vi "IOC_LV_Panel1.vi"() -> ()   [LabVIEW 2016]
uses:
  <vilib>/Utility/miscctls.llb/LVPointTypeDef.ctl
  <vilib>/Instr/_visa.llb/VISA Configure Serial Port (Instr).vi
panel:
  in  "Boolean":bool
  in  "Baud rate":u64=230400
  in  "COM Port":refnum<visa-resource-name>
  in  "ms":i32=50
  in  "Analog Input Gain":u8 format="%.0b"
  in  "New Address":u8=170
  in  "set Address":bool
  in  "set sn":bool
  in  "New S/N":u32 format="%08x"
  out "S/N":u32 format="%08x"
  out "CPU Clock":u32=170 caption="Clock" format="%.0f [sec]"
  in  "Address":u8=170
  out "value 2":u8=170 caption="value"
  in  "index 2":u8=99 caption="index[0..99]" max=99 step=1
  in  "set scratch":bool
  in  "value":u8=170
  in  "index[0..99]":u8=99 max=99
  out "disable?":bool
  out "gui_refresh":bool
  in  "DigTimeout":u16=170 caption="Digital Timeout[sec]"
  in  "DIGITAL_IO":T1={"DIG_PORT_0 [0..7] (P4)"=[FALSE, FALSE, FALSE, FALSE, FALSE, FALSE, FALSE, FALSE], "DIG_PORT_1 [8..15] (P5)"=[FALSE, FALSE, FALSE, FALSE, FALSE, FALSE, FALSE, FALSE], "DIG_PORT_2 [16..23]  (P3)"=[FALSE, FALSE, FALSE, FALSE, FALSE, FALSE, FALSE, FALSE], "DIG_PORT_3  [24..31]  (P2)"=[FALSE, FALSE, FALSE, FALSE, FALSE, FALSE, FALSE, FALSE], "DIG_PORT_4   [32..39]  (P6)"=[FALSE, FALSE, FALSE, FALSE, FALSE, FALSE, FALSE, FALSE], "DIG_PORT_5  [40..47]  (P7)"=[FALSE, FALSE, FALSE, FALSE, FALSE, FALSE, FALSE, FALSE]} caption="Digital In/Out"
  in  "scan":bool
  in  "Table Control":string[][](table)
  out "user msg":string
  out "Chart":T2(graph)
  in  "AOUT0[%]":dbl(knob) scale=0.0..100.0
  in  "AOUT1[%]":dbl(knob) scale=0.0..100.0
  in  "counter":i32
  in  "stop":bool
  # "Module Setup"
  # "Module Setup"
  # "Virtual Address Setup"
  # "Read Module Data"
  # "Serial Number Setup"
  # "Get Scratch Memory"
  # "Set Scratch Memory"
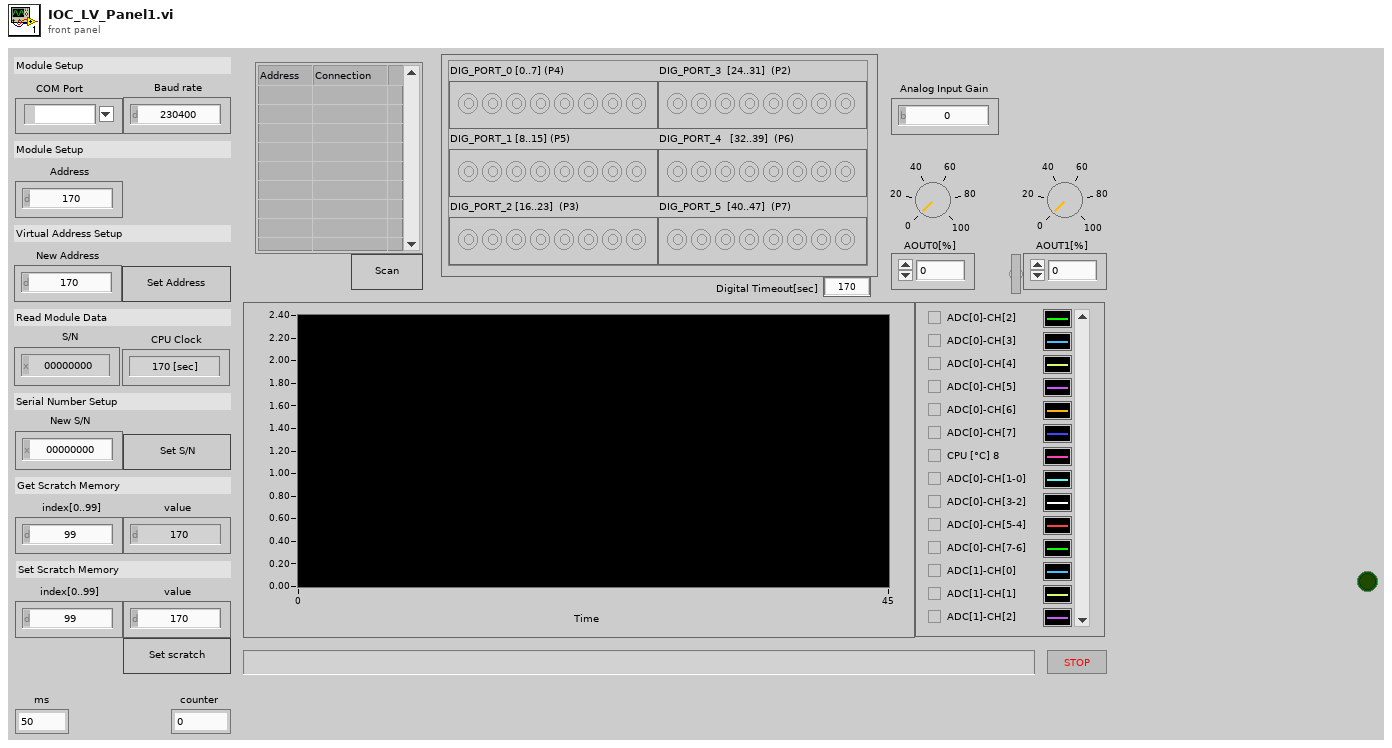
[diagram p1: front panel]
types:
  T1 = cluster{"DIG_PORT_0 [0..7] (P4)":bool[], "DIG_PORT_1 [8..15] (P5)":bool[], "DIG_PORT_2 [16..23]  (P3)":bool[], "DIG_PORT_3  [24..31]  (P2)":bool[], "DIG_PORT_4   [32..39]  (P6)":bool[], "DIG_PORT_5  [40..47]  (P7)":bool[]}
  T2 = cluster{"[0]":sgl, "[1]":sgl, "[2]":sgl, "[3]":sgl, "[4]":sgl, "[5]":sgl, "[6]":sgl, "[7]":sgl, "[8]":sgl, "[9]":sgl, "[10]":sgl, "[11]":sgl, "[12]":sgl, "[13]":sgl, "[14]":sgl, "[15]":sgl, "[16]":sgl, "[17]":sgl, "[18]":sgl, "[19]":sgl, "[20]":sgl}
  T3 = typedef "LVPointTypeDef.ctl" = cluster{"Horizontal":i16, "Vertical":i16}
  T4 = cluster{"ADDRESS":u8, "AOUT CHANNEL":u8, "AOUT value":u16}
  T5 = cluster{"ADDRESS[0.255]":u8, "AIN CHANNEL[0..7]":u8, "gain":u8}
  T6 = cluster{"DIG_PORT_0 [0..7] (P4)":bool[], "DIG_PORT_1 [8..15] (P5)":bool[], "DIG_PORT_2 [16..23]  (P3)":bool[], "DIG_PORT_3  [23..31]  (P2)":bool[], "DIG_PORT_4   [32..39]  (P6)":bool[], "DIG_PORT_5  [40..47]  (P7)":bool[]}
  T7 = cluster{"Address":u8, "index of element":i32, i16, "DigTimeout":u16}
  T8 = cluster{"Address":u8, i32, i16, "DigTimeout":u16}
  T9 = typedef "lveventtype.ctl" = enum32{"Null", "Timeout", "Annotation Menu Selection", "Annotation Menu Selection?", "App Instance Close", "App Instance Close?", "Autoscale Range Change", "Bookmark Info Change", "Cell Edit", "Cell Edit?", "Cursor Grab", "Cursor Grab?", "Cursor Menu Selection", "Cursor Menu Selection?", "Cursor Move", "Cursor Release", "Data Change", "Direction Change", "Display State Change", "Drag Ended", "Drag Enter", "Drag Leave", "Drag Over", "Drag Source Update", "Drag Starting", "Drag Starting?", "Drop", "Exec State Change", "Key Down", "Key Down?", "Key Repeat", "Key Repeat?", "Key Up", "Listbox Double Click", "Menu Activation?", "Menu Selection (App)", "Menu Selection? (App)", "Menu Selection (User)", "Mouse Down", "Mouse Down?", "Mouse Enter", "Mouse Leave", "Mouse Move", "Mouse Up", "Mouse Wheel", "NI Security User Change (App)", "Pane Size", "Panel Close", "Panel Close?", "Panel Resize", "Plot Attribute Change", "Scale Range Change", "Shortcut Menu Activation?", "Shortcut Menu Selection (App)", "Shortcut Menu Selection? (App)", "Shortcut Menu Selection (User)", "Tree Double Click", "Tree Drag", "Tree Drag?", "Tree Drop", "Tree Drop?", "Tree Item Close", "Tree Item Close?", "Tree Item Open", "Tree Item Open?", "User Event", "Value Change"}
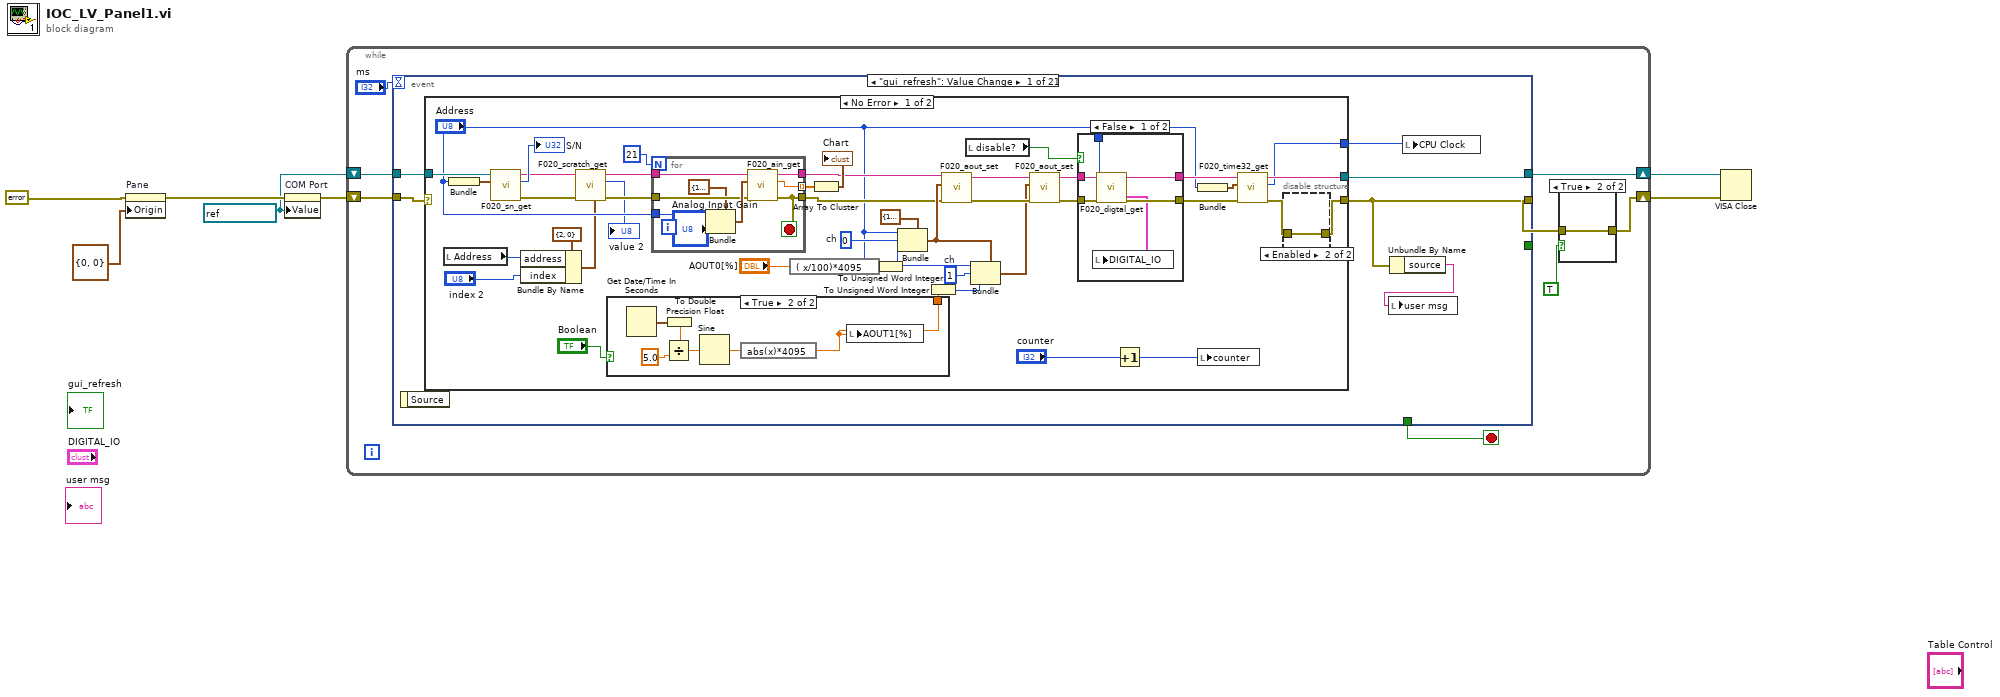
[diagram p0: block diagram]
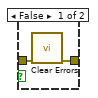
[diagram p2: hidden frame]
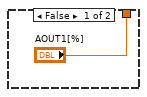
[diagram p3: hidden frame]
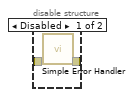
[diagram p4: hidden frame]
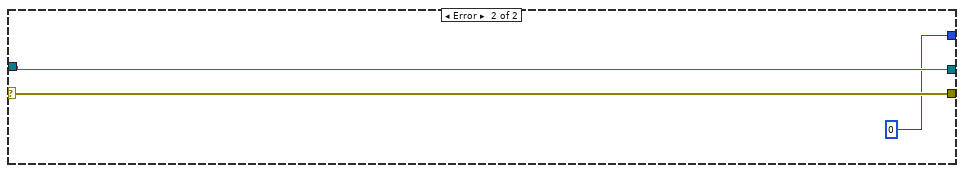
[diagram p6: hidden frame]
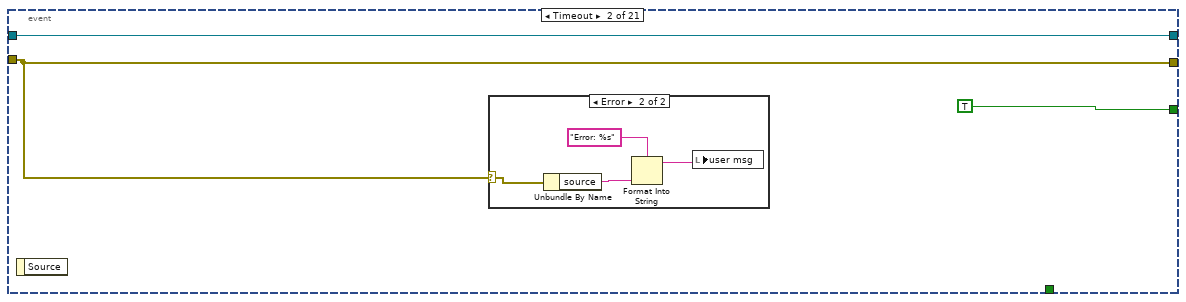
[diagram p7: hidden frame]
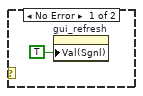
[diagram p8: hidden frame]
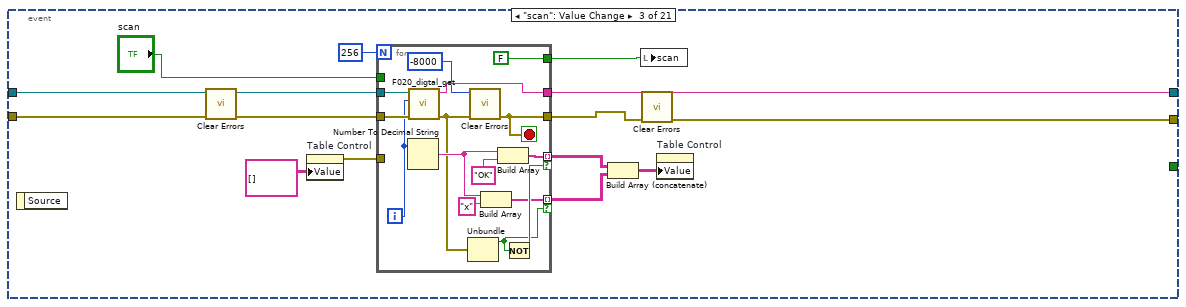
[diagram p9: hidden frame]
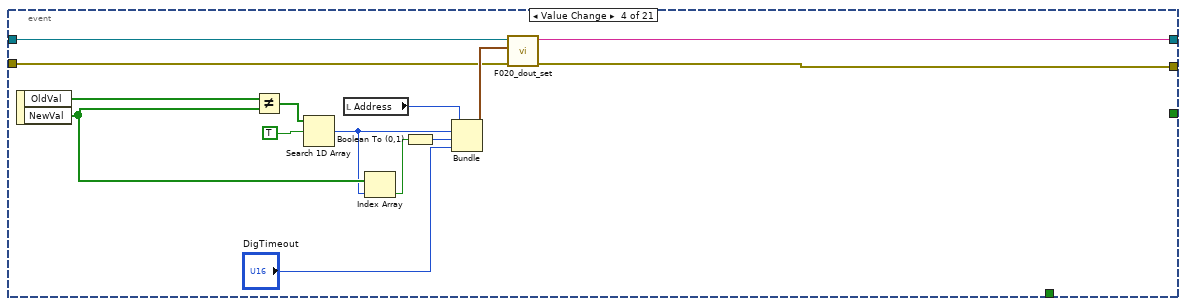
[diagram p10: hidden frame]
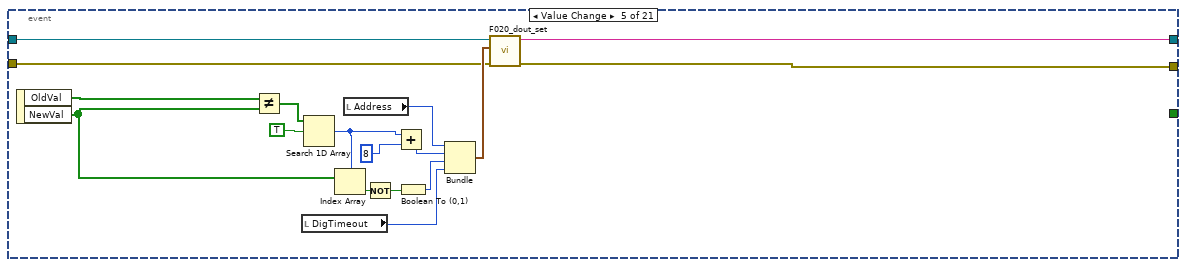
[diagram p11: hidden frame]
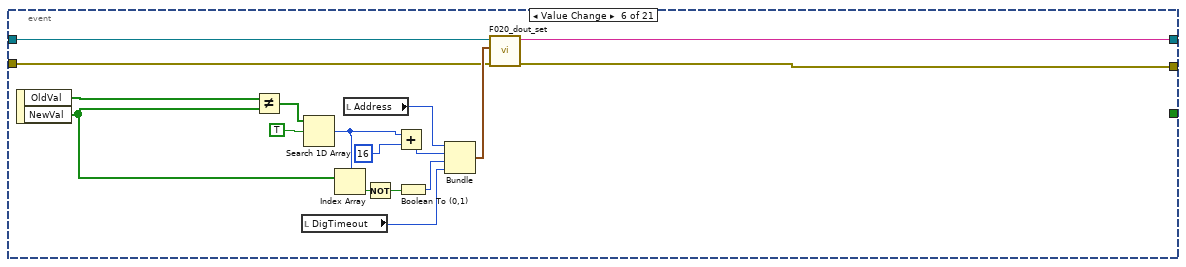
[diagram p12: hidden frame]
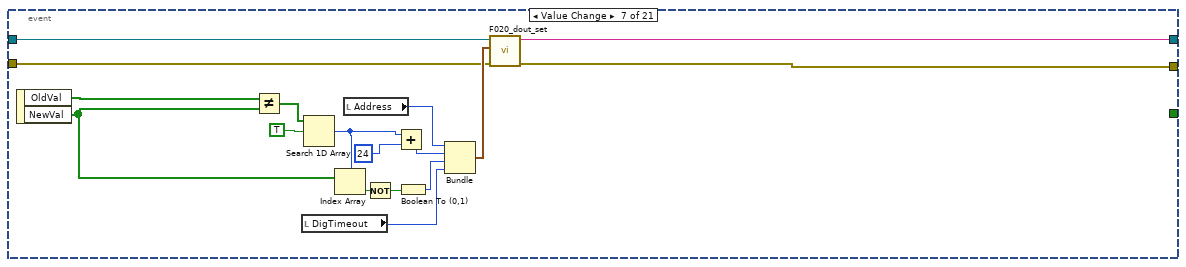
[diagram p13: hidden frame]
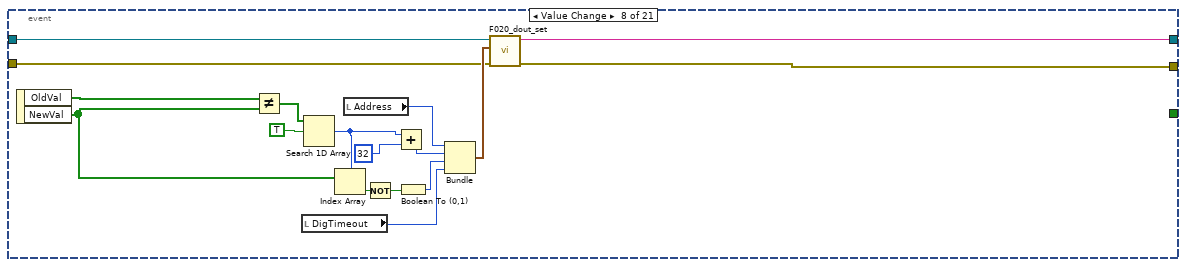
[diagram p14: hidden frame]
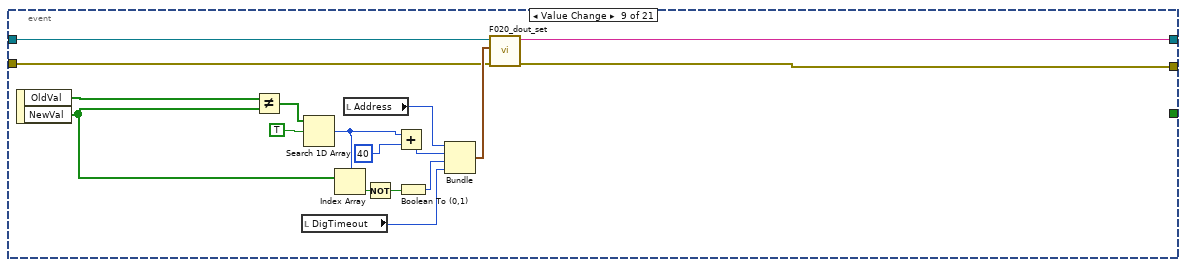
[diagram p15: hidden frame]
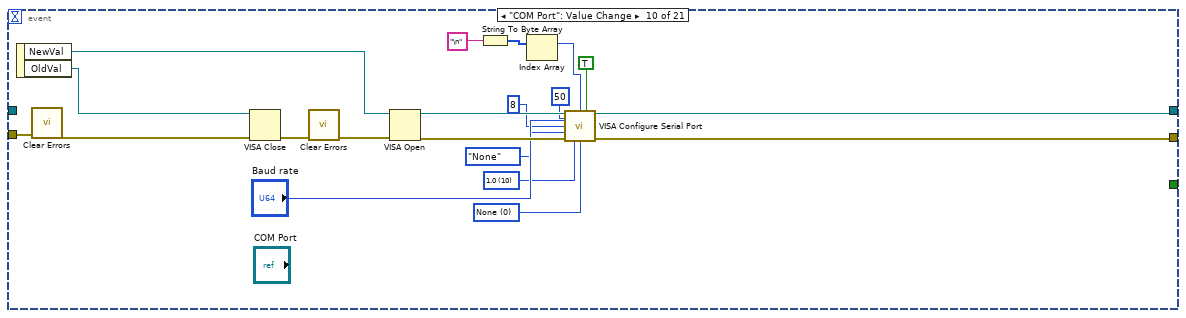
[diagram p16: hidden frame]
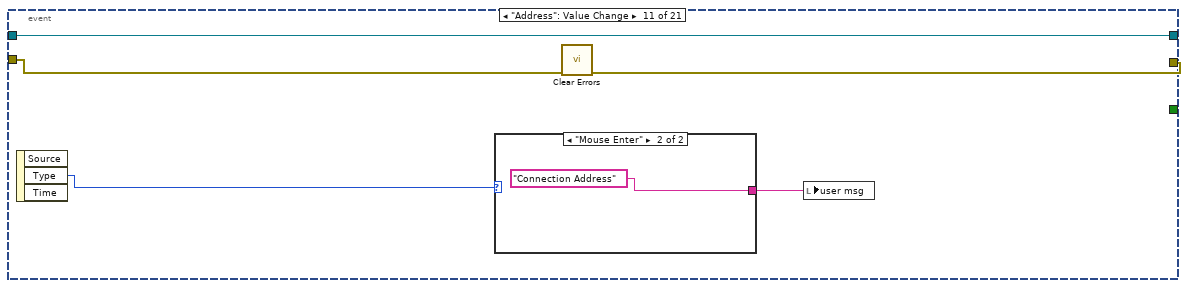
[diagram p17: hidden frame]
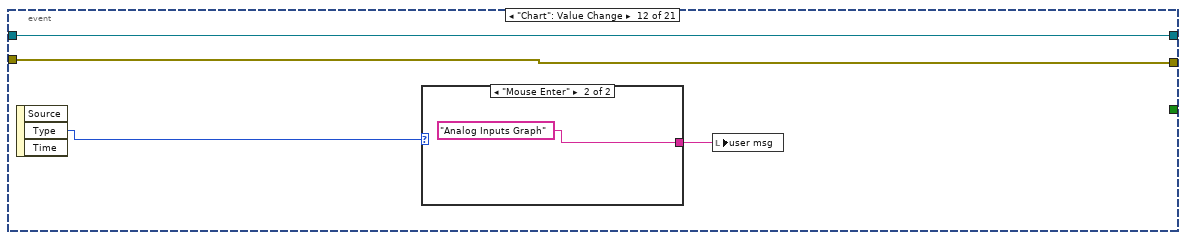
[diagram p19: hidden frame]
diagram:
  w1 = refnum<visa-resource-name> refnum ("Value (Signaling)")
  n1 = property on="Pane" class="Pane"(error in=errorcluster {"status"=TRUE, "code"=0, "source"="Undefined COM Port"} ("error in (no error)"), "Origin"=T3 {"Horizontal"=0, "Vertical"=0}) -> (error out=w2:errorcluster)  [unwired: 1 in, 1 out]
  n2 = property on="COM Port" class="VISAName"(error in=w2, "Value"=w1) -> (error out=w5:errorcluster)  [unwired: 1 in, 1 out]
  n3 = while {
    shift-right: [w14] -> w7
    shift-left: w1 -> [w13]
    shift-right: [w9] -> w6
    shift-left: w5 -> [w10]
    stop <- w15 stop-if-true
    n4 = event shown="[0] \"gui_refresh\": Value Change" {
      selector: _ -> [_ _ _ _ _ _ _ _ _ _ _ _ _ _ _ _ _ _ _ _ _]
      dyn-events: _ -> [_ _ _ _ _ _ _ _ _ _ _ _ _ _ _ _ _ _ _ _ _]
      timeout: "ms" -> [_ _ _ _ _ _ _ _ _ _ _ _ _ _ _ _ _ _ _ _ _]
      tunnel: [_ _ _ _ _ _ _ _ _ _ _ _ _ _ _ _ "stop" _ _ _ _] -> w15
      tunnel: [w23 w101 w118 w139 w158 w175 w192 w209 w226 w251 w259 w264 w269 w277 w286 w294 w300 w305 w310 w315 w321] -> w14
      tunnel: w13 -> [w24 w101 w119 w140 w159 w176 w193 w210 w227 _ w259 w264 w271 w279 w288 w296 w300 w305 w310 w315 w321]
      tunnel: [w20 w100 w109 w138 w150 w167 w184 w201 w218 w249 w257 w261 w270 w278 w287 w295 w299 w302 w307 w312 w317] -> w11
      tunnel: w10 -> [w22 w100 w120 w136 w151 w168 w185 w202 w219 w239 w258 w261 w272 w280 w289 w297 w299 w302 w307 w312 w317]
      tunnel: [_ TRUE ("Value (Signaling)") _ _ _ _ _ _ _ _ _ _ _ _ _ _ _ _ _ _ _] -> _
      event "gui_refresh": Value Change {
        n5 = event-data() -> ()  [unwired: 1 in, 1 out]
        n6 = case shown="No Error" w22 {
          selector: w22 -> [_ w97]
          tunnel: w24 -> [w43 w98]
          tunnel: [w29 w97] -> w20
          tunnel: [w51 w98] -> w23
          tunnel: [w49 u32 0 ("RUNTIME out")] -> w21
          frame No Error {
            w59 = u8 1  # ch
            w64 = u8 0  # ch
            n7 = local read "Address"() -> (w35:u8)
            n8 = Bundle("Address"="Address") -> (w41:cluster{"Address":u8})  [unwired: 1 in]
            n9 = call "F020_sn_get.vi"("Cluster"=w41, "COM in"=w43) -> ("error out"=w37:errorcluster, "SN"=→"S/N":u32, "COM out"=w39:string)  [unwired: 7 in]
            n10 = Bundle By Name(cluster=cluster{"address":u32, "index":u32} {"address"=2, "index"=0} ("Cluster"), "address"=w35, "index"="index 2") -> (w33:cluster{"address":u32, "index":u32})
            n11 = call "F020_scratch_get.vi"("error in"=w37, "Cluster"=w33, "COM in"=w39) -> ("error out"=w36:errorcluster, "value"=→"value 2":u32, "COM out"=w38:string)  [unwired: 6 in]
            n12 = case shown="True" "Boolean" {
              tunnel: ["AOUT1[%]" w69] -> w26
              frame False {
              }
              frame True {
                n13 = Get Date/Time In Seconds() -> (seconds since 1Jan1904=w74:timestamp)
                n14 = To Double Precision Float(number=w74) -> (double precision float=w72:dbl)
                n15 = Divide(x=w72, y=5.0) -> (x/y=w70:dbl)
                n16 = Sine(x=w70) -> (sin(x)=w73:dbl)
                n17 = expression code="abs(x)*4095"(w73) -> (w69:dbl)
                n18 = local write "AOUT1[%]"(w69) -> ()
              }
            }
            n19 = for {
              N: 21 -> [_]
              tunnel: [w95] -> w57
              tunnel: w38 -> [w94]
              tunnel: [w91] -> w66 mode=indexing
              tunnel: [w90] -> w56
              tunnel: "Address" -> [w89]
              tunnel: w36 -> [w88]
              i -> [w92]
              stop <- w90 stop-if-true
              n20 = Bundle(cluster=T5 {"ADDRESS[0.255]"=170, "AIN CHANNEL[0..7]"=0, "gain"=0} ("Cluster"), "ADDRESS[0.255]"=w89, "AIN CHANNEL[0..7]"=w92, "gain"="Analog Input Gain") -> (w93:T5)
              n21 = call "F020_ain_get.vi"("error in"=w88, "Cluster"=w93, "COM in"=w94) -> ("error out"=w90:errorcluster, "ain"=w91:sgl, "COM out"=w95:string)  [unwired: 6 in]
            }
            n22 = expression code="( x/100)*4095"("AOUT0[%]") -> (w47:dbl)
            n23 = Array To Cluster(array=w66) -> (cluster=→"Chart":T2)
            n24 = To Unsigned Word Integer(number=w47) -> (unsigned 16bit integer=w46:u16)
            n25 = Bundle(cluster=T4 {"ADDRESS"=123, "AOUT CHANNEL"=1, "AOUT value"=2048} ("Cluster"), "ADDRESS"="Address", "AOUT CHANNEL"=w64, "AOUT value"=w46) -> (w61:T4)
            n26 = To Unsigned Word Integer(number=w26) -> (unsigned 16bit integer=w45:u16)
            n27 = call "F020_aout_set.vi"("error in"=w56, "Cluster"=w61, "COM in"=w57) -> ("error out"=w62:errorcluster, "COM out"=w63:string)  [unwired: 7 in]
            n28 = local read "disable?"() -> (w48:bool)
            n29 = Bundle(cluster=w61, "ADDRESS"="Address", "AOUT CHANNEL"=w59, "AOUT value"=w45) -> (w58:T4)
            n30 = call "F020_aout_set.vi"("error in"=w62, "Cluster"=w58, "COM in"=w63) -> ("error out"=w55:errorcluster, "COM out"=w54:string)  [unwired: 7 in]
            n31 = case shown="False" w48 {
              tunnel: w55 -> [w83 w84]
              tunnel: w54 -> [w82 w85]
              tunnel: [w81 w84] -> w53
              tunnel: [w80 w85] -> w52
              tunnel: "Address" -> [w79 _]
              frame False {
                n32 = call "F020_digtal_get.vi"("error in"=w83, "ADDRESS"=w79, "COM in"=w82) -> ("error out"=w81:errorcluster, "COM out"=w80:string, "DIGITAL_IO"=w78:T6)  [unwired: 4 in, 2 out]
                n33 = local write "DIGITAL_IO"(w78) -> ()
              }
              frame True {
              }
            }
            n34 = Increment(x="counter") -> (x+1=w27:i32)
            n35 = Bundle("Address"="Address") -> (w50:cluster{"Address":u8})  [unwired: 1 in]
            n36 = local write "counter"(w27) -> ()
            n37 = call "F020_time32_get.vi"("error in"=w53, "Cluster"=w50, "COM in"=w52) -> ("error out"=w30:errorcluster, "RUNTIME out"=w49:u32, "COM out"=w51:string)  [unwired: 6 in]
            n38 = disable-structure shown="Enabled" {
              disable-tunnel: w30 -> [w76 w77]
              disable-tunnel: [w75 w77] -> w29
              frame Disabled {
                n39 = call <vilib>:"Simple Error Handler.vi"("error in (no error)"=w76) -> ("error out"=w75:errorcluster)  [unwired: 4 in, 4 out]
              }
              frame Enabled {
              }
            }
          }
          frame Error {
          }
        }
        n40 = Unbundle By Name(w20) -> ("source"=w19:string)
        n41 = local write "user msg"(w19) -> ()
        n42 = local write "CPU Clock"(w21) -> ()
      }
      event Timeout {
        n43 = event-data() -> ()  [unwired: 1 in, 1 out]
        n44 = case shown="Error" w100 {
          selector: w100 -> [_ w103]
          frame No Error {
            n45 = property on="gui_refresh" class="Bool (strict)"("Val(Sgnl)"=TRUE ("Value (Signaling)")) -> ()  [unwired: 2 in, 2 out]
          }
          frame Error {
            n46 = Unbundle By Name(w103) -> ("source"=w105:string)
            n47 = Format Into String(format string="Error: %s", w105) -> (resulting string=w104:string)  [unwired: 2 in, 1 out]
            n48 = local write "user msg"(w104) -> ()
          }
        }
      }
      event "scan": Value Change {
        n49 = event-data() -> ()  [unwired: 1 in, 1 out]
        n50 = call <vilib>:"Clear Errors.vi"("error in (no error)"=w120) -> ("error out"=w110:errorcluster)  [unwired: 5 in, 1 out]
        n51 = property on="Table Control" class="Tbl (strict)"("Value"=string[][] [] ("Table Control")) -> (error out=w112:errorcluster)  [unwired: 2 in, 1 out]
        n52 = for {
          N: 256 -> [_]
          tunnel: w119 -> [w134]
          tunnel: [w133] -> w118
          tunnel: [w130] -> w116 mode=indexing if=w131
          tunnel: [w126] -> w115 mode=indexing if=w125
          tunnel: w110 -> [w135]
          tunnel: [w122] -> w111
          tunnel: w112 -> [_]
          tunnel: "scan" -> [_]
          tunnel: [FALSE ("scan")] -> w107
          i -> [w132]
          stop <- w122 stop-if-true
          n53 = Number To Decimal String(number=w132) -> (decimal integer string=w127:string)  [unwired: 1 in]
          n54 = call "F020_digtal_get.vi"("error in"=w135, "ADDRESS"=w132, "COM in"=w134) -> ("error out"=w124:errorcluster, "COM out"=w133:string)  [unwired: 4 in, 3 out]
          n55 = Unbundle(w124) -> ("status"=w125:bool)  [unwired: 2 out]
          n56 = call <vilib>:"Clear Errors.vi"("error in (no error)"=w124, "specific error code to clear (0: all)"=-8000) -> ("error out"=w122:errorcluster)  [unwired: 4 in, 1 out]
          n57 = Build Array(w127, "x" ("source")) -> (w126:string[])
          n58 = Build Array(w127, "OK" ("source")) -> (w130:string[])
          n59 = Not(x=w125) -> (.not. x?=w131:bool)
        }
        n60 = Build Array (concatenate)(w116, w115) -> (w114:string[][])
        n61 = local write "scan"(w107) -> ()
        n62 = call <vilib>:"Clear Errors.vi"("error in (no error)"=w111) -> ("error out"=w109:errorcluster)  [unwired: 5 in, 1 out]
        n63 = property on="Table Control" class="Tbl (strict)"("Value"=w114) -> ()  [unwired: 2 in, 2 out]
      }
      event "DIGITAL_IO.DIG_PORT_0 [0..7] (P4)": Value Change {
        n64 = event-data() -> ("OldVal"=w149:bool[], "NewVal"=w145:bool[])  [unwired: 1 in]
        n65 = Not Equal?(x=w149, y=w145) -> (x != y?=w148:bool[])
        n66 = Search 1D Array(1D array=w148, element=TRUE) -> (index of element=w144:i32)  [unwired: 1 in]
        n67 = local read "Address"() -> (w146:u8)
        n68 = Index Array(array=w145, index=w144) -> (element=w143:bool)
        n69 = Boolean To (0,1)(Boolean=w143) -> (0, 1=w142:i16)
        n70 = Bundle("Address"=w146, "index of element"=w144, w142, "DigTimeout"="DigTimeout") -> (w141:T7)  [unwired: 1 in]
        n71 = call "F020_dout_set.vi"("error in"=w136, "Cluster"=w141, "COM in"=w140) -> ("error out"=w138:errorcluster, "COM out"=w139:string)  [unwired: 7 in]
      }
      event "DIGITAL_IO.DIG_PORT_1 [8..15] (P5)": Value Change {
        n72 = event-data() -> ("OldVal"=w166:bool[], "NewVal"=w162:bool[])  [unwired: 1 in]
        n73 = Not Equal?(x=w166, y=w162) -> (x != y?=w165:bool[])
        n74 = local read "DigTimeout"() -> (w152:u16)
        n75 = Search 1D Array(1D array=w165, element=TRUE) -> (index of element=w155:i32)  [unwired: 1 in]
        n76 = Index Array(array=w162, index=w155) -> (element=w161:bool)
        n77 = local read "Address"() -> (w163:u8)
        n78 = Not(x=w161) -> (.not. x?=w153:bool)
        n79 = Add(x=w155, y=i16 8) -> (x+y=w154:i32)
        n80 = Boolean To (0,1)(Boolean=w153) -> (0, 1=w156:i16)
        n81 = Bundle("Address"=w163, w154, w156, "DigTimeout"=w152) -> (w160:T8)  [unwired: 1 in]
        n82 = call "F020_dout_set.vi"("error in"=w151, "Cluster"=w160, "COM in"=w159) -> ("error out"=w150:errorcluster, "COM out"=w158:string)  [unwired: 7 in]
      }
      event "DIGITAL_IO.DIG_PORT_2 [16..23]  (P3)": Value Change {
        n83 = event-data() -> ("OldVal"=w183:bool[], "NewVal"=w179:bool[])  [unwired: 1 in]
        n84 = Not Equal?(x=w183, y=w179) -> (x != y?=w182:bool[])
        n85 = local read "DigTimeout"() -> (w169:u16)
        n86 = Search 1D Array(1D array=w182, element=TRUE) -> (index of element=w172:i32)  [unwired: 1 in]
        n87 = Index Array(array=w179, index=w172) -> (element=w178:bool)
        n88 = local read "Address"() -> (w180:u8)
        n89 = Not(x=w178) -> (.not. x?=w170:bool)
        n90 = Add(x=w172, y=i16 16) -> (x+y=w171:i32)
        n91 = Boolean To (0,1)(Boolean=w170) -> (0, 1=w173:i16)
        n92 = Bundle("Address"=w180, w171, w173, "DigTimeout"=w169) -> (w177:T8)  [unwired: 1 in]
        n93 = call "F020_dout_set.vi"("error in"=w168, "Cluster"=w177, "COM in"=w176) -> ("error out"=w167:errorcluster, "COM out"=w175:string)  [unwired: 7 in]
      }
      event "DIGITAL_IO.DIG_PORT_3  [24..31]  (P2)": Value Change {
        n94 = event-data() -> ("OldVal"=w200:bool[], "NewVal"=w196:bool[])  [unwired: 1 in]
        n95 = Not Equal?(x=w200, y=w196) -> (x != y?=w199:bool[])
        n96 = local read "DigTimeout"() -> (w186:u16)
        n97 = Search 1D Array(1D array=w199, element=TRUE) -> (index of element=w189:i32)  [unwired: 1 in]
        n98 = Index Array(array=w196, index=w189) -> (element=w195:bool)
        n99 = local read "Address"() -> (w197:u8)
        n100 = Not(x=w195) -> (.not. x?=w187:bool)
        n101 = Add(x=w189, y=i16 24) -> (x+y=w188:i32)
        n102 = Boolean To (0,1)(Boolean=w187) -> (0, 1=w190:i16)
        n103 = Bundle("Address"=w197, w188, w190, "DigTimeout"=w186) -> (w194:T8)  [unwired: 1 in]
        n104 = call "F020_dout_set.vi"("error in"=w185, "Cluster"=w194, "COM in"=w193) -> ("error out"=w184:errorcluster, "COM out"=w192:string)  [unwired: 7 in]
      }
      event "DIGITAL_IO.DIG_PORT_4   [32..39]  (P6)": Value Change {
        n105 = event-data() -> ("OldVal"=w217:bool[], "NewVal"=w213:bool[])  [unwired: 1 in]
        n106 = Not Equal?(x=w217, y=w213) -> (x != y?=w216:bool[])
        n107 = local read "DigTimeout"() -> (w203:u16)
        n108 = Search 1D Array(1D array=w216, element=TRUE) -> (index of element=w206:i32)  [unwired: 1 in]
        n109 = Index Array(array=w213, index=w206) -> (element=w212:bool)
        n110 = local read "Address"() -> (w214:u8)
        n111 = Not(x=w212) -> (.not. x?=w204:bool)
        n112 = Add(x=w206, y=i16 32) -> (x+y=w205:i32)
        n113 = Boolean To (0,1)(Boolean=w204) -> (0, 1=w207:i16)
        n114 = Bundle("Address"=w214, w205, w207, "DigTimeout"=w203) -> (w211:T8)  [unwired: 1 in]
        n115 = call "F020_dout_set.vi"("error in"=w202, "Cluster"=w211, "COM in"=w210) -> ("error out"=w201:errorcluster, "COM out"=w209:string)  [unwired: 7 in]
      }
      event "DIGITAL_IO.DIG_PORT_5  [40..47]  (P7)": Value Change {
        n116 = event-data() -> ("OldVal"=w234:bool[], "NewVal"=w230:bool[])  [unwired: 1 in]
        n117 = Not Equal?(x=w234, y=w230) -> (x != y?=w233:bool[])
        n118 = local read "DigTimeout"() -> (w220:u16)
        n119 = Search 1D Array(1D array=w233, element=TRUE) -> (index of element=w223:i32)  [unwired: 1 in]
        n120 = Index Array(array=w230, index=w223) -> (element=w229:bool)
        n121 = local read "Address"() -> (w231:u8)
        n122 = Not(x=w229) -> (.not. x?=w221:bool)
        n123 = Add(x=w223, y=i16 40) -> (x+y=w222:i32)
        n124 = Boolean To (0,1)(Boolean=w221) -> (0, 1=w224:i16)
        n125 = Bundle("Address"=w231, w222, w224, "DigTimeout"=w220) -> (w228:T8)  [unwired: 1 in]
        n126 = call "F020_dout_set.vi"("error in"=w219, "Cluster"=w228, "COM in"=w227) -> ("error out"=w218:errorcluster, "COM out"=w226:string)  [unwired: 7 in]
      }
      event "COM Port": Value Change {
        w243 = u16 10 items=["1.0"=10, "1.5"=15, "2.0"=20] ("stop bits (10: 1 bit)")
        w242 = u16 0 items=["None", "XON/XOFF", "RTS/CTS", "XON/XOFF & RTS/CTS", "DTR/DSR", "XON/XOFF & DTR/DSR"] ("flow control (0:none)")
        n127 = event-data() -> ("NewVal"=w240:refnum<visa-resource-name>, "OldVal"=w241:refnum<visa-resource-name>)  [unwired: 1 in]
        n128 = call <vilib>:"Clear Errors.vi"("error in (no error)"=w239) -> ("error out"=w238:errorcluster)  [unwired: 5 in, 1 out]
        n129 = VISA Close(VISA resource name=w241, error in (no error)=w238) -> (error out=w254:errorcluster)
        n130 = call <vilib>:"Clear Errors.vi"("error in (no error)"=w254) -> ("error out"=w253:errorcluster)  [unwired: 5 in, 1 out]
        n131 = VISA Open(error in (no error)=w253, VISA resource name=w240) -> (VISA resource name=w252:refnum<visa-resource-name>, error out=w250:errorcluster)  [unwired: 3 in]
        n132 = String To Byte Array(string="\n") -> (unsigned byte array=w236:u8[])
        n133 = Index Array(array=w236) -> (element=w235:u8)  [unwired: 1 in]
        n134 = call-poly "VISA Configure Serial Port"("VISA resource name"=w252, "timeout (10sec)"=u32 50, "termination char\n(0xA = '\\n' = LF)"=w235, "Enable Termination\nChar (T)"=TRUE ("Enable Termination\nChar (T)"), "baud rate (9600)"="Baud rate", "data bits (8)"=u16 8, "parity (0:none)"=enum16{"None", "Odd", "Even", "Mark", "Space"}."None", "error in (no error)"=w250, "stop bits (10: 1 bit)"=w243, "flow control (0:none)"=w242) -> ("VISA resource name out"=w251:refnum<visa-resource-name>, "error out"=w249:errorcluster)  [unwired: 4 in]
      }
      event "Address": Value Change {
        n135 = event-data() -> ("Type"=w255:T9)  [unwired: 1 in, 2 out]
        n136 = case shown="\"Mouse Enter\"" w255 {
          tunnel: [_ "Connection Address" ("user msg")] -> w256
          frame Default {
          }
          frame "Mouse Enter" {
          }
        }
        n137 = call <vilib>:"Clear Errors.vi"("error in (no error)"=w258) -> ("error out"=w257:errorcluster)  [unwired: 5 in, 1 out]
        n138 = local write "user msg"(w256) -> ()
      }
      event "Chart": Value Change {
        n139 = event-data() -> ("Type"=w262:T9)  [unwired: 1 in, 2 out]
        n140 = case shown="\"Mouse Enter\"" w262 {
          tunnel: [_ "Analog Inputs Graph" ("user msg")] -> w263
          frame Default {
          }
          frame "Mouse Enter" {
          }
        }
        n141 = local write "user msg"(w263) -> ()
      }
      event "set Address": Value Change {
        n142 = event-data() -> ()  [unwired: 1 in, 3 out]
        n143 = local read "Address"() -> (w266:u8)
        n144 = Bundle By Name(cluster=cluster{"Old Address":u8, "New Address":u8} {"Old Address"=170, "New Address"=0} ("Cluster"), "Old Address"=w266, "New Address"="New Address") -> (w273:cluster{"Old Address":u8, "New Address":u8})
        n145 = call "F020_vaddr_set.vi"("error in"=w272, "Cluster"=w273, "COM in"=w271) -> ("error out"=w270:errorcluster, "COM out"=w269:string)  [unwired: 7 in]
      }
      event "set sn": Value Change {
        n146 = event-data() -> ()  [unwired: 1 in, 3 out]
        n147 = local read "Address"() -> (w276:u8)
        n148 = Bundle By Name(cluster=cluster{"address":u32, "SN":u32} {"address"=2, "SN"=15728641} ("Cluster"), "address"=w276, "SN"="New S/N") -> (w281:cluster{"address":u32, "SN":u32})
        n149 = call "F020_sn_set.vi"("error in"=w280, "Cluster"=w281, "COM in"=w279) -> ("error out"=w278:errorcluster, "COM out"=w277:string)  [unwired: 7 in]
      }
      event "set scratch": Value Change {
        n150 = event-data() -> ()  [unwired: 1 in, 1 out]
        n151 = local read "Address"() -> (w285:u8)
        n152 = Bundle By Name(cluster=cluster{"address":u32, "index":u32, "value":u32} {"address"=2, "index"=100, "value"=0} ("Cluster"), "address"=w285, "index"="index[0..99]", "value"="value") -> (w290:cluster{"address":u32, "index":u32, "value":u32})
        n153 = call "F020_scratch_set.vi"("error in"=w289, "Cluster"=w290, "COM in"=w288) -> ("error out"=w287:errorcluster, "COM out"=w286:string)  [unwired: 7 in]
      }
      event "CPU Clock": Value Change {
        n154 = event-data() -> ()  [unwired: 1 in, 3 out]
        n155 = local read "CPU Clock"() -> (w291:u32)
        n156 = local read "Address"() -> (w292:u8)
        n157 = Bundle By Name(cluster=cluster{"ADDRESS":u8, "time_U32":u32} {"ADDRESS"=170, "time_U32"=170} ("Cluster"), "ADDRESS"=w292, "time_U32"=w291) -> (w298:cluster{"ADDRESS":u8, "time_U32":u32})
        n158 = call "F020_time32_set.vi"("error in"=w297, "Cluster"=w298, "COM in"=w296) -> ("error out"=w295:errorcluster, "COM out"=w294:string)  [unwired: 6 in, 1 out]
      }
      event "stop": Value Change {
        n159 = event-data() -> ()  [unwired: 1 in, 1 out]
      }
      event "CPU Clock": Mouse Enter; "CPU Clock": Mouse Leave {
        n160 = event-data() -> ("Type"=w303:T9)  [unwired: 1 in, 2 out]
        n161 = case shown="\"Mouse Enter\"" w303 {
          tunnel: [_ "32-bit Second  Counter" ("user msg")] -> w304
          frame Default {
          }
          frame "Mouse Enter" {
          }
        }
        n162 = local write "user msg"(w304) -> ()
      }
      event "COM Port": Mouse Enter; Mouse Leave {
        n163 = event-data() -> ("Type"=w309:T9)  [unwired: 1 in, 2 out]
        n164 = case shown="\"Mouse Enter\"" w309 {
          tunnel: [_ "Serial Port" ("user msg")] -> w308
          frame Default {
          }
          frame "Mouse Enter" {
          }
        }
        n165 = local write "user msg"(w308) -> ()
      }
      event "Address": Mouse Enter; "Address": Mouse Leave {
        n166 = event-data() -> ("Type"=w314:T9)  [unwired: 1 in, 2 out]
        n167 = case shown="Default" w314 {
          tunnel: [_ "Module Address" ("user msg")] -> w313
          frame Default {
          }
          frame "Mouse Enter" {
          }
        }
        n168 = local write "user msg"(w313) -> ()
      }
      event "DIGITAL_IO": Mouse Enter; "DIGITAL_IO": Mouse Leave {
        n169 = event-data() -> ("Type"=w320:T9)  [unwired: 1 in, 3 out]
        n170 = case shown="Default" w320 {
          tunnel: ["Read Enable" ("user msg") "Write Enable" ("user msg")] -> w319
          tunnel: [_ TRUE ("OK Button 2")] -> w318
          frame Default {
          }
          frame "Mouse Enter" {
          }
        }
        "disable?" <- w318
        n171 = local write "user msg"(w319) -> ()
      }
    }
    n172 = case shown="True" TRUE {
      tunnel: w11 -> [w17 w18]
      tunnel: [w16 w18] -> w9
      frame False {
        n173 = call <vilib>:"Clear Errors.vi"("error in (no error)"=w17) -> ("error out"=w16:errorcluster)  [unwired: 5 in, 1 out]
      }
      frame True {
      }
    }
  }
  n174 = VISA Close(VISA resource name=w7, error in (no error)=w6) -> ()  [unwired: 1 out]
